vi "JLINKARM Close.vi"(8 "error in (no error)":errorcluster) -> (0 "error out":errorcluster)   [LabVIEW 2020, in "JLinkARM.lvlib"]
doc: "JLINKARMDLL_API void JLINKARM_Close (void);"
uses:
  Lib/JLinkARM.lvlib
  JLinkARM.dll
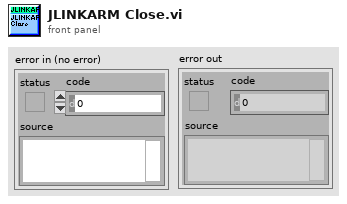
[diagram p1: front panel]
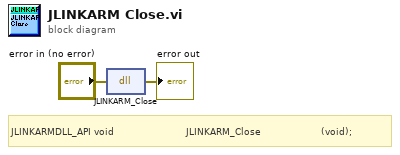
[diagram p0: block diagram]
diagram:
  # "JLINKARMDLL_API void                        JLINKARM_Close                    (void);"
  n1 = dll-call lib="C:/Users/anybody/Desktop/JLinkARM.*" fn="JLINKARM_Close"(error in="error in (no error)") -> (error out=→"error out":errorcluster)  [unwired: 3 in, 1 out]
